vi "MH_InitChannels.vi"(11 "nchannels":i32) -> (2 "SetInpChan":T2[](array[typedef]), 3 "Channels":T1[](array[typedef]) {"DeadTime" min=800 max=160000 step=1; "Edge" items=["falling", "rising"]; "Offset" min=-100000 max=100000 step=80; "Level" min=-1200 max=1200 step=1})   [LabVIEW 2017]
uses:
  Types/MH_SetInpChanData.ctl
  Types/MH_SetInpChanCmds.ctl
  Types/MH_InputChannel.ctl
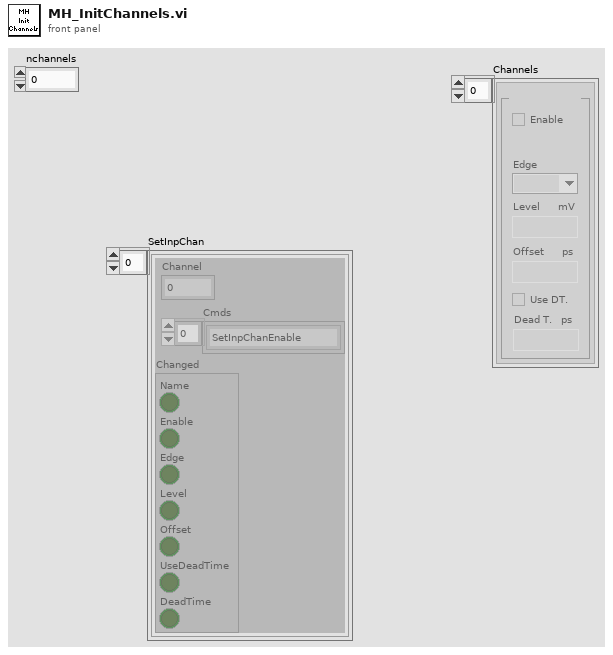
[diagram p1: front panel]
types:
  T1 = typedef "MH_InputChannel.ctl" = cluster{"Name":string, "Enable":bool, "Edge":i32, "Level":i32, "Offset":i32, "UseDeadTime":bool, "DeadTime":i32}
  T2 = typedef "MH_SetInpChanData.ctl" = cluster{"Channel":i32, "Cmds":T3[], "Changed":cluster{"Name":bool, "Enable":bool, "Edge":bool, "Level":bool, "Offset":bool, "UseDeadTime":bool, "DeadTime":bool}}
  T3 = typedef "MH_SetInpChanCmds.ctl" = enum16{"SetInpChanEnable", "SetInpChanOffset", "SetInpChanDeadTime", "SetInpChanTrg"}
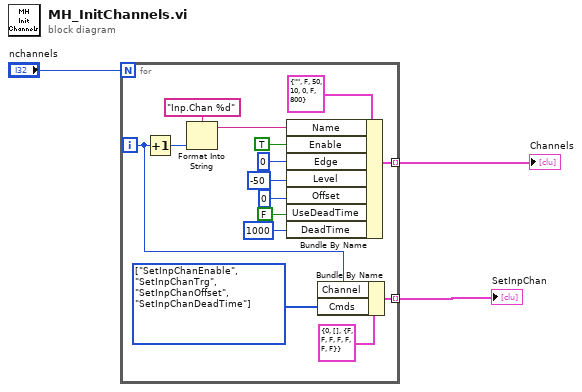
[diagram p0: block diagram]
diagram:
  n1 = for {
    N: "nchannels" -> [_]
    tunnel: [w18] -> w1 mode=indexing
    tunnel: [w5] -> w2 mode=indexing
    i -> [w6]
    w4 = T3[] [enum."SetInpChanEnable", enum."SetInpChanTrg", enum."SetInpChanOffset", enum."SetInpChanDeadTime"] items=["SetInpChanEnable", "SetInpChanOffset", "SetInpChanDeadTime", "SetInpChanTrg"]
    n2 = Increment(x=w6) -> (x+1=w11:i32)
    n3 = Format Into String(format string="Inp.Chan %d", w11) -> (resulting string=w16:string)  [unwired: 2 in, 1 out]
    n4 = Bundle By Name(cluster=T1 {"Name"="", "Enable"=FALSE, "Edge"=50, "Level"=10, "Offset"=0, "UseDeadTime"=FALSE, "DeadTime"=800} ("Channel"), "Name"=w16, "Enable"=TRUE, "Edge"=0 ("Offset"), "Level"=-50 ("CFDZeroX"), "Offset"=0 ("CFDLevel"), "UseDeadTime"=FALSE, "DeadTime"=1000) -> (w18:T1)
    n5 = Bundle By Name(cluster=T2 {"Channel"=0, "Cmds"=[], "Changed"={"Name"=FALSE, "Enable"=FALSE, "Edge"=FALSE, "Level"=FALSE, "Offset"=FALSE, "UseDeadTime"=FALSE, "DeadTime"=FALSE}}, "Channel"=w6, "Cmds"=w4) -> (w5:T2)
  }
  "SetInpChan" <- w2
  "Channels" <- w1
